vi "ex7-6.vi"   [LabVIEW 2013]
uses:
  <vilib>/NXT/Block Support/NXT_InputPort.ctl
  <vilib>/NXT/Block Support/NXT_OutputPort.ctl
  <vilib>/NXT/Dual Mode Library/Sensors/EV3_Ultrasonic_CM.vi
  <vilib>/NXT/NXTIO Xnodes/NXTIONodeSubVIs/NXTMoveMotors.vi
  <vilib>/NXT/Subs/LVHSConnector.ctl
  <vilib>/NXT/NXTIO Xnodes/AddressXNode/NXTIOAddress.xnode
  <vilib>/NXT/NXTIO Xnodes/NXTIOXNode/NXTIO.xnode
  <vilib>/NXT/LegoClasses/BrickReference/BrickReference.lvclass
types:
  T1 = typedef "NXT_OutputPort.ctl" = u8
  T2 = typedef "NXT_InputPort.ctl" = u32
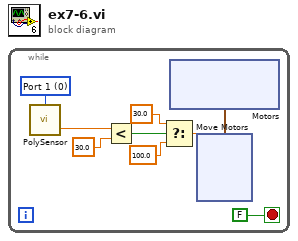
[diagram p0: block diagram]
diagram:
  n1 = while {
    stop <- FALSE stop-if-true
    w6 = T2 0 items=["Port 1", "Port 2", "Port 3", "Port 4"] ("Port (Port 1)")
    n2 = call-poly <vilib>:"PolySensor.vi"("Port (Port 1)"=w6) -> ("Centimeters"=w8:sgl)  [unwired: 2 in, 1 out]
    n3 = Less?(x=w8, y=sgl 30.0) -> (x < y?=w9:bool)
    n4 = Select(t=30.0, s=w9, f=100.0) -> (s? t:f=w5:dbl)
    n5 = xnode "Motors"() -> ("Motor"=w2:cluster{"Port":T1, "Port":T1})
    n6 = xnode "Move Motors"("Power/Speed 1"=w5, "Motors"=w2) -> ()  [unwired: 2 in, 1 out]
  }
